vi "Add Error.vi"(8 "error in (no error)":errorcluster, 9 "String to Append":string, 10 "Error":T1, 11 "Insert Error":bool=TRUE) -> (0 "error out":errorcluster)   [LabVIEW 2021, in "Template_Common.lvlib"]
doc: "This VI will insert a custome error message. This wrapper is designed to be inlined to minimize overhead when there is no error. It calls an error core VI that should not be inlined to minimize memory impact."
uses:
  Template_Common.lvlib
  Typedef/Errors.ctl
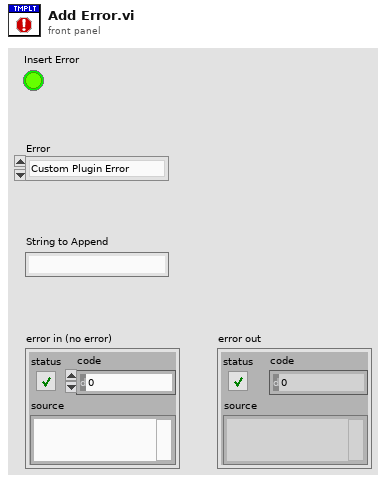
[diagram p1: front panel]
types:
  T1 = typedef "Template_Common.lvlib/Errors.ctl" = enum16{"Custom Plugin Error"}
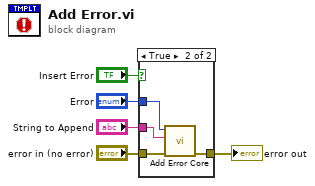
[diagram p0: block diagram]
diagram:
  n1 = case shown="True" "Insert Error" {
    tunnel: [w6 w7] -> w4
    tunnel: "error in (no error)" -> [w6 w8]
    tunnel: "Error" -> [_ w10]
    tunnel: "String to Append" -> [_ w9]
    frame False {
    }
    frame True {
      n2 = call "Add Error Core.vi"("error in (no error)"=w8, "String to Append"=w9, "Error"=w10) -> ("error out"=w7:errorcluster)  [unwired: 8 in]
    }
  }
  "error out" <- w4
